vi "Configure GB Low Limit.vi"(8 "error in (no error)":errorcluster, 9 "Lo Limit [Ohm]":dbl=0.001 min=0.0 max=0.1 step=0.0001 format="%.1p", 10 "Step":T1=1 min=1 max=99 step=1, 11 "VISA resource name":refnum<visa-resource-name>) -> (0 "error out":errorcluster, 3 "VISA resource name out":refnum<visa-resource-name>)   [LabVIEW 2025, in "Chroma 19572.lvlib"]
uses:
  <instrlib>/Chroma 19572/Chroma 19572.lvlib
  <instrlib>/Chroma 19572/Public/Utility/Type Def/steps--numeric.ctl
panel:
  # "Configure GB Low Limit"
  # "0=OFF\n0,1 to 100 mOhm"
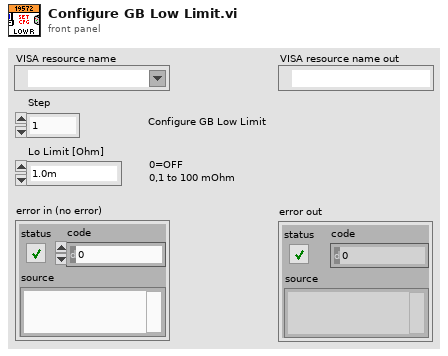
[diagram p1: front panel]
types:
  T1 = typedef "Chroma 19572.lvlib/steps--numeric.ctl" = u8
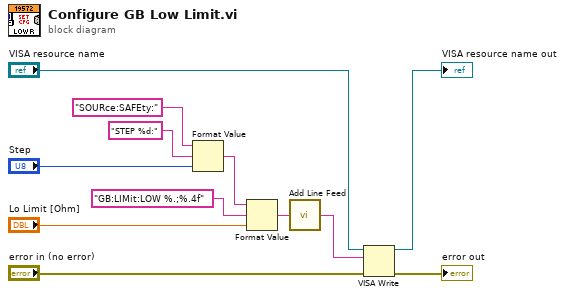
[diagram p0: block diagram]
diagram:
  n1 = Format Value(string ("")="SOURce:SAFEty:", format string="STEP %d:", value (0)="Step") -> (output string=w1:string)
  n2 = Format Value(string ("")=w1, format string="GB:LIMit:LOW %.;%.4f", value (0)="Lo Limit [Ohm]") -> (output string=w7:string)
  n3 = call <instrlib>:"Add Line Feed.vi"("Command string"=w7) -> ("Concatenated string"=w2:string)  [unwired: 4 in]
  n4 = VISA Write(VISA resource name="VISA resource name", write buffer=w2, error in (no error)="error in (no error)") -> (VISA resource name out=→"VISA resource name out":refnum<visa-resource-name>, error out=→"error out":errorcluster)  [unwired: 1 out]
